vi "LSX Get Controller Factor.vi"(0 "lLSID":i32, 1 "pdR":dbl, 5 "pdX":dbl, 7 "pdY":dbl, 9 "pdZ":dbl, 11 "error in (no error)":errorcluster) -> (3 "pdR out":dbl, 4 "function return":i32, 6 "pdX out":dbl, 8 "pdY out":dbl, 10 "pdZ out":dbl, 15 "error out":errorcluster)   [LabVIEW 2018, in "Tango.lvlib"]
doc: "TANGOAPI int TANGOCALL LSX_GetControllerFactor (int lLSID, double *pdX, double *pdY, double *pdZ, double *pdR);"
uses:
  Tango.lvlib
  SubVIs/Tango_DLL.dll
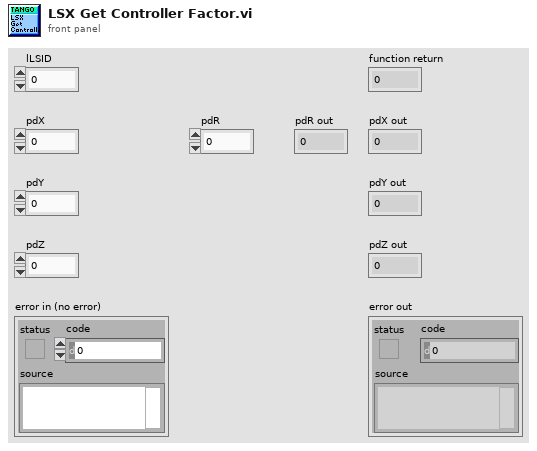
[diagram p1: front panel]
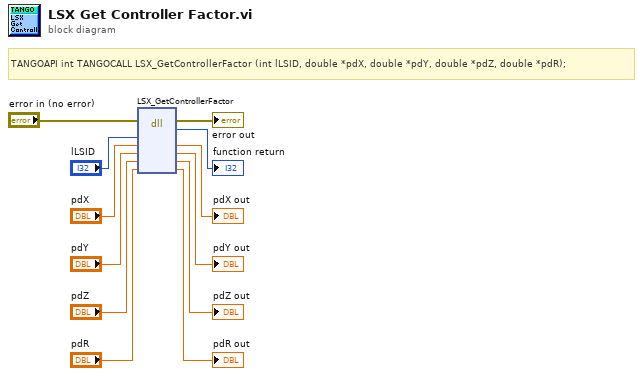
[diagram p0: block diagram]
diagram:
  # "TANGOAPI int TANGOCALL LSX_GetControllerFactor (int lLSID, double *pdX, double *pdY, double *pdZ, double *pdR);"
  n1 = dll-call lib="C:/Users/Familie/Documents/LabviewIX81/lib/TANGO Stage/SubVIs/Tango_DLL.*" fn="LSX_GetControllerFactor"(error in="error in (no error)", "lLSID"="lLSID", "pdX"="pdX", "pdY"="pdY", "pdZ"="pdZ", "pdR"="pdR") -> (error out=→"error out":errorcluster, →"function return":i32, "pdX"=→"pdX out":dbl, "pdY"=→"pdY out":dbl, "pdZ"=→"pdZ out":dbl, "pdR"=→"pdR out":dbl)  [unwired: 3 in, 1 out]
